vi "Parameters SLM.vi"(1 "Action 2":u16(ring) items=["ParamAuto", "ParamUser"], 2 "Action":u16(ring) items=["Save", "Load"], 13 "Array":string[](array[string])) -> ()   [LabVIEW 2012]
uses:
  <vilib>/Utility/file.llb/Write To Spreadsheet File (DBL).vi
  <vilib>/Utility/file.llb/Read From Spreadsheet File (DBL).vi
  <vilib>/Utility/VariantDataType/VariantType.lvlib
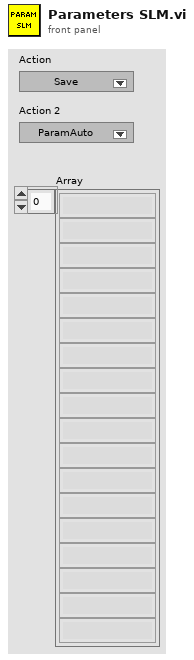
[diagram p1: front panel]
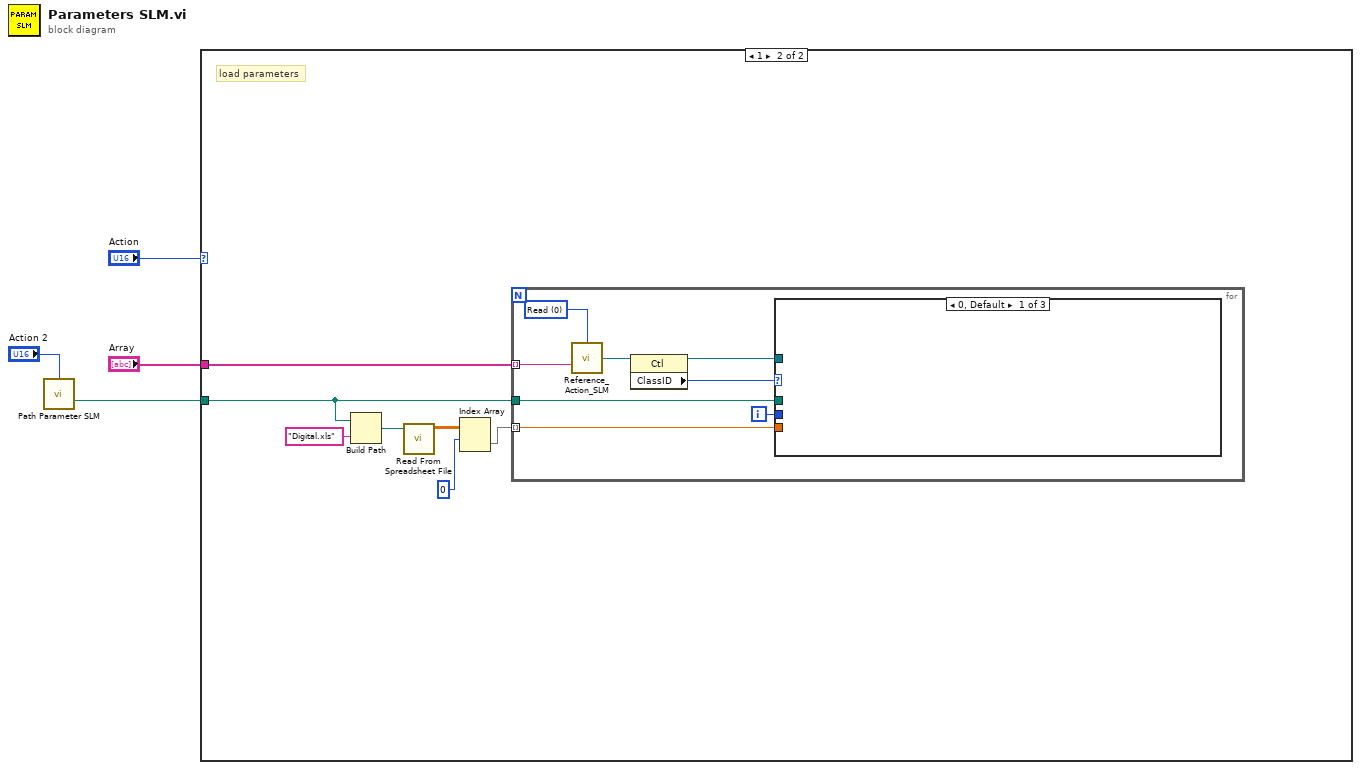
[diagram p0: block diagram]
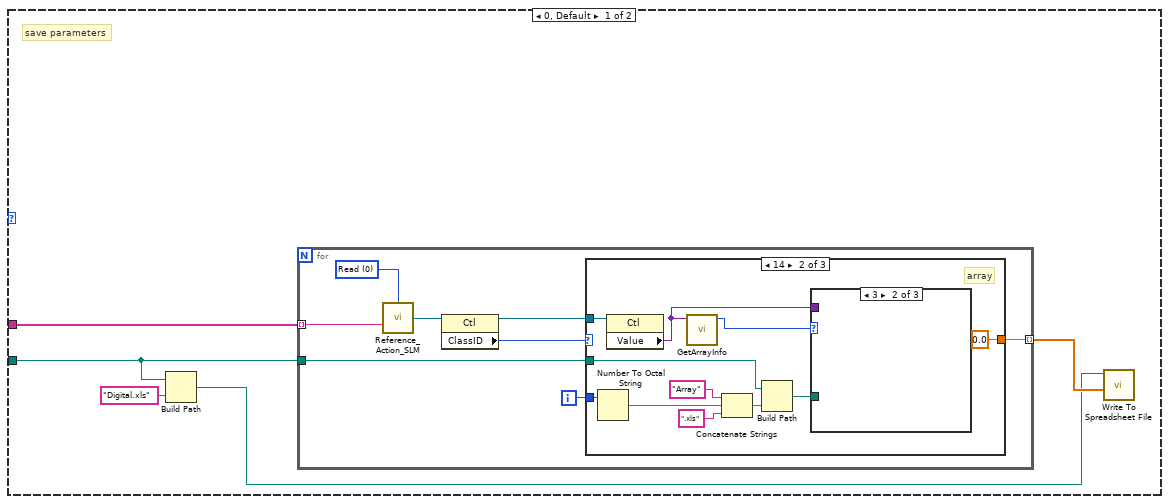
[diagram p2: hidden frame]
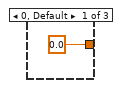
[diagram p3: hidden frame]
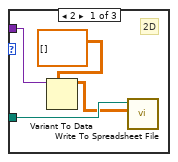
[diagram p4: hidden frame]
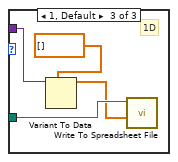
[diagram p5: hidden frame]
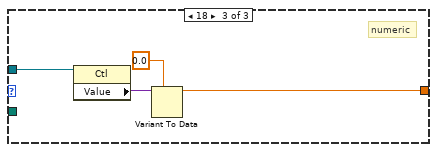
[diagram p6: hidden frame]
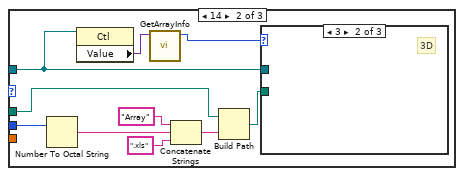
[diagram p7: hidden frame]
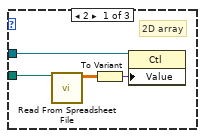
[diagram p8: hidden frame]
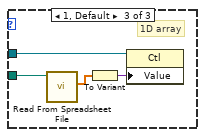
[diagram p9: hidden frame]
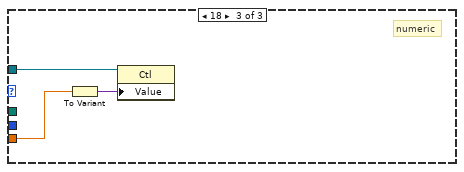
[diagram p10: hidden frame]
diagram:
  n1 = call "Path Parameter SLM.vi"("Action"="Action 2") -> ("appended path"=w2:path)  [unwired: 14 in]
  n2 = case shown="1" "Action" {
    tunnel: "Array" -> [w9 w48]
    tunnel: w2 -> [w6 w43]
    frame 0, Default {
      # "save parameters"
      n3 = Build Path(base path=w6, name or relative path="Digital.xls") -> (appended path=w5:path)
      n4 = for {
        tunnel: w9 -> [w17] mode=indexing
        tunnel: [w13] -> w8 mode=indexing
        tunnel: w6 -> [w11]
        i -> [w10]
        w16 = u16 0 items=["Read", "Initialize"] ("Action")
        n5 = call "Reference_Action_SLM.vi"("Action"=w16, "Control Name"=w17) -> ("Ref OUT"=w15:refnum<vi>)  [unwired: 11 in, 2 out]
        n6 = property class="Ctl"(reference=w15) -> (reference out=w14:refnum<vi>, "ClassID"=w12:u32)  [unwired: 1 in, 1 out]
        n7 = case shown="14" w12 {
          tunnel: w14 -> [_ w29 w41]
          tunnel: [0.0 ("type") 0.0 ("type") w38] -> w13
          tunnel: w11 -> [_ w25 _]
          tunnel: w10 -> [_ w24 _]
          frame 0, Default {
          }
          frame 14 {
            # "array"
            n8 = Number To Octal String(2:w24) -> (0:w27:string)  [unwired: 1 in]
            n9 = property class="Ctl"(reference=w29) -> ("Value"=w20:variant)  [unwired: 1 in, 2 out]
            n10 = call <vilib>:"GetArrayInfo.vi"("Variant"=w20) -> ("NDims"=w19:i32)  [unwired: 7 in, 3 out]
            n11 = Concatenate Strings("Array" ("name or relative path"), w27, ".xls" ("name or relative path")) -> (w26:string)
            n12 = Build Path(base path=w25, name or relative path=w26) -> (appended path=w23:path)
            n13 = case shown="3" w19 {
              tunnel: w23 -> [w33 _ w37]
              tunnel: w20 -> [w32 _ w36]
              frame 2 {
                # "2D"
                n14 = Variant To Data(type=dbl[][] [], Variant=w32) -> (data=w30:dbl[][])  [unwired: 1 in, 1 out]
                n15 = call-poly <vilib>:"Write To Spreadsheet File.vi"("2D data"=w30, "file path (dialog if empty)"=w33) -> ()  [unwired: 6 in, 1 out]
              }
              frame 3 {
              }
              frame 1, Default {
                # "1D"
                n16 = Variant To Data(type=dbl[] [], Variant=w36) -> (data=w34:dbl[])  [unwired: 1 in, 1 out]
                n17 = call-poly <vilib>:"Write To Spreadsheet File.vi"("1D data"=w34, "file path (dialog if empty)"=w37) -> ()  [unwired: 6 in, 1 out]
              }
            }
          }
          frame 18 {
            # "numeric"
            n18 = property class="Ctl"(reference=w41) -> ("Value"=w39:variant)  [unwired: 1 in, 2 out]
            n19 = Variant To Data(type=0.0, Variant=w39) -> (data=w38:dbl)  [unwired: 1 in, 1 out]
          }
        }
      }
      n20 = call-poly <vilib>:"Write To Spreadsheet File.vi"("1D data"=w8, "file path (dialog if empty)"=w5) -> ()  [unwired: 6 in, 1 out]
    }
    frame 1 {
      # "load parameters"
      n21 = Build Path(base path=w43, name or relative path="Digital.xls") -> (appended path=w42:path)
      n22 = call-poly <vilib>:"Read From Spreadsheet File.vi"("file path (dialog if empty)"=w42) -> ("all rows"=w47:dbl[][])  [unwired: 6 in, 4 out]
      n23 = Index Array(array=w47, index (row)=0) -> (element=w45:dbl[])  [unwired: 1 in]
      n24 = for {
        tunnel: w48 -> [w56] mode=indexing
        tunnel: w43 -> [w50]
        tunnel: w45 -> [w49] mode=indexing
        i -> [w51]
        w55 = u16 0 items=["Read", "Initialize"] ("Action")
        n25 = call "Reference_Action_SLM.vi"("Action"=w55, "Control Name"=w56) -> ("Ref OUT"=w54:refnum<vi>)  [unwired: 11 in, 2 out]
        n26 = property class="Ctl"(reference=w54) -> (reference out=w53:refnum<vi>, "ClassID"=w52:u32)  [unwired: 1 in, 1 out]
        n27 = case shown="0, Default" w52 {
          tunnel: w53 -> [_ w59 w77]
          tunnel: w51 -> [_ w60 _]
          tunnel: w50 -> [_ w66 _]
          tunnel: w49 -> [_ _ w75]
          frame 0, Default {
          }
          frame 14 {
            n28 = Number To Octal String(2:w60) -> (0:w63:string)  [unwired: 1 in]
            n29 = property class="Ctl"(reference=w59) -> ("Value"=w58:variant)  [unwired: 1 in, 2 out]
            n30 = call <vilib>:"GetArrayInfo.vi"("Variant"=w58) -> ("NDims"=w57:i32)  [unwired: 7 in, 3 out]
            n31 = Concatenate Strings("Array" ("name or relative path"), w63, ".xls" ("name or relative path")) -> (w61:string)
            n32 = Build Path(base path=w66, name or relative path=w61) -> (appended path=w65:path)
            n33 = case shown="3" w57 {
              tunnel: w65 -> [w70 _ w74]
              tunnel: w59 -> [w69 _ w73]
              frame 2 {
                # "2D array"
                n34 = call-poly <vilib>:"Read From Spreadsheet File.vi"("file path (dialog if empty)"=w70) -> ("all rows"=w68:dbl[][])  [unwired: 6 in, 4 out]
                n35 = To Variant(anything=w68) -> (Variant=w67:variant)
                n36 = property class="Ctl"(reference=w69, "Value"=w67) -> ()  [unwired: 1 in, 2 out]
              }
              frame 3 {
                # "3D"
              }
              frame 1, Default {
                # "1D array"
                n37 = call-poly <vilib>:"Read From Spreadsheet File.vi"("file path (dialog if empty)"=w74) -> ("first row"=w72:dbl[])  [unwired: 6 in, 4 out]
                n38 = To Variant(anything=w72) -> (Variant=w71:variant)
                n39 = property class="Ctl"(reference=w73, "Value"=w71) -> ()  [unwired: 1 in, 2 out]
              }
            }
          }
          frame 18 {
            # "numeric"
            n40 = To Variant(anything=w75) -> (Variant=w76:variant)
            n41 = property class="Ctl"(reference=w77, "Value"=w76) -> ()  [unwired: 1 in, 2 out]
          }
        }
      }
    }
  }
